vi "HIL.vi"(0 "System no.":i32=1 min=1 max=4 step=1, 2 "DeviceID to set":i32[](array[numeric]), 3 "Value":i32[](array[numeric]), 5 "error in":errorcluster, 6 "DeviceLED":i32[](array[numeric])) -> (14 "Controller error":bool, 19 "error out":errorcluster)   [LabVIEW 2026]
doc: "Sets the state of the LEDs of a Human Interface Device (HID) and queries ERR?. \"LED\" stands for hardware-dependent output, which can be an LED or a force-feedback actuator. See controller user manual for details. Controller error is TRUE if selected system reports error code which is not 0."
panel:
  # "Sets the state of the LEDs of a Human Interface Device (HID) and queries ERR?. \"LED\" \nstands for hardware-dependent output, which can be an LED or a force-feedback \nactuator. See controller User Manual for details."
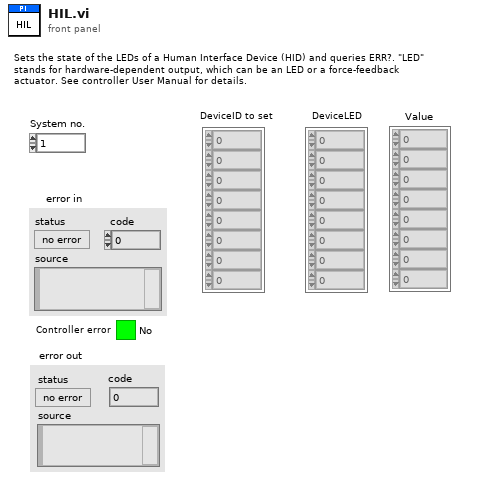
[diagram p1: front panel]
types:
  T1 = enum16{"Disable error check", "Force error check", "Use global settings"}
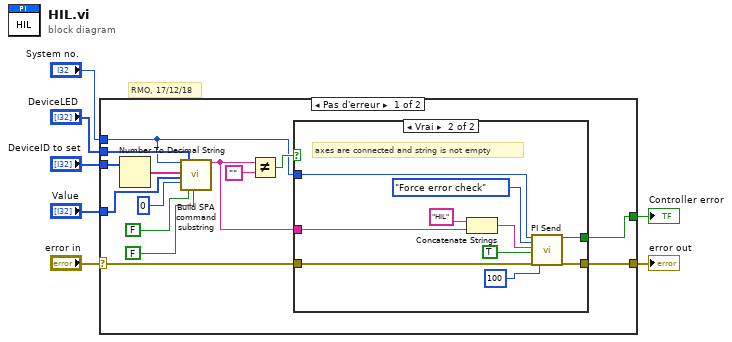
[diagram p0: block diagram]
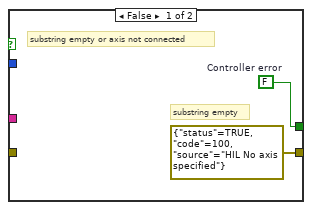
[diagram p2: hidden frame]
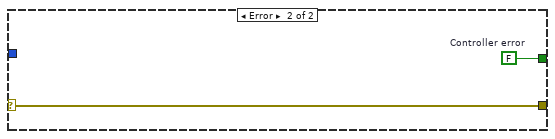
[diagram p3: hidden frame]
diagram:
  # "RMO, 17/12/18"
  n1 = case shown="Pas d'erreur" "error in" {
    selector: "error in" -> [w9 w35]
    tunnel: [w21 w35] -> w7
    tunnel: "Value" -> [w18 _]
    tunnel: "System no." -> [w15 _]
    tunnel: "DeviceID to set" -> [w13 _]
    tunnel: "DeviceLED" -> [w17 _]
    tunnel: [w8 w34] -> w1
    frame No Error {
      n2 = Number To Decimal String(number=w13) -> (decimal integer string=w12:string[])  [unwired: 1 out]
      n3 = call "Build SPA command substring.vi"("System no."=w15, "Axes to set"=w12, "Parameter values"=w18, "No. of digits"=i16 0, "Parameter number"=w17, "Parameter no. format \n(Decimal: FALSE)"=FALSE ("Parameter no. format \n(Decimal: FALSE)"), "Parameter format \n(Num.: FALSE)"=FALSE ("Parameter format \n(Num.: FALSE)")) -> ("SPA command substring"=w19:string)  [unwired: 3 in, 9 out]
      n4 = Not Equal?(x=w19, y="") -> (x != y?=w16:bool)
      n5 = case shown="Vrai" w16 {
        tunnel: w19 -> [_ w32]
        tunnel: [errorcluster {"status"=TRUE, "code"=100, "source"="HIL No axis specified"} ("error out") w26] -> w21
        tunnel: w9 -> [_ w29]
        tunnel: w15 -> [_ w28]
        tunnel: [w22 w24] -> w8
        frame False {
          w22 = FALSE  # Controller error
          # "substring empty"
          # "substring empty or axis not connected"
        }
        frame True {
          # "axes are connected and string is not empty"
          n6 = Concatenate Strings("HIL", w32) -> (w30:string)
          n7 = call "PI Send.vi"("System no."=w28, "Error check settings"=T1."Force error check", "String to send"=w30, "Attach termination char.?"=TRUE ("Attach Linefeed?"), "error in"=w29, "Delay before error check (ms)"=u32 100 ("milliseconds to wait")) -> ("Controller error"=w24:bool, "error out"=w26:errorcluster)  [unwired: 12 out]
        }
      }
    }
    frame Error {
      w34 = FALSE  # Controller error
    }
  }
  "error out" <- w7
  "Controller error" <- w1
